vi "TempStrainRecord.vi"() -> ()   [LabVIEW 2024]
uses:
  <vilib>/Analysis/baseanly.llb/Mean (DBL).vi
  <vilib>/DAQmx/create/channels.llb/DAQmx Create Channel (AI-Temperature-Thermocouple).vi
  <vilib>/DAQmx/configure/trigger.llb/DAQmx Start Trigger (Digital Edge).vi
  <vilib>/Utility/TDMS File Viewer/NI_TDMS File Viewer.lvlib
  <vilib>/Analysis/NI_AALBase.lvlib
panel:
  in  "stop":bool
  out "status":bool
  out "DAQ error out":errorcluster caption="error out"
  out "Temp loop counter":i32
  out "mean 2":dbl format="%0.2f"
  out "mean 3":dbl format="%0.2f"
  out "mean 4":dbl format="%0.2f"
  out "mean 5":dbl format="%0.2f"
  out "data 5":dynamicdata(graph) caption="data"
  out "data 4":dynamicdata(graph) caption="data"
  out "mean 0":dbl format="%0.2f"
  out "data 3":dynamicdata(graph) caption="data"
  out "data 2":dynamicdata(graph) caption="data"
  out "data 1":dynamicdata(graph) caption="data"
  out "data 0":dynamicdata(graph) caption="data"
  out "mean 1":dbl format="%0.2f"
  out "Temperature TDMS error out":errorcluster
  out "TCP warning out":errorcluster
  out "TDMS Close error out":errorcluster
  out "TCP counter":i32
  out "Complete String after 'Bytes to read'":string
  out "Bytes to read (hex)":string
  out "Bytes to read (dec)":i32
  out "Qty of Optical Lines":string
  out "LineNumber":string
  out "Date":string
  out "OpticalLineNumber":string[](array[string])
  out "Qty of FBG's":string[](array[string])
  out "System Status":string[][](array[string])
  out "Peak Wavelengths":string[][](array[string])
  out "Peak Powers":string[][](array[string])
  out "Time":string
  in  "Address":string="127.0.0.1"
  in  "Port":u16=2055 min=1025 step=1
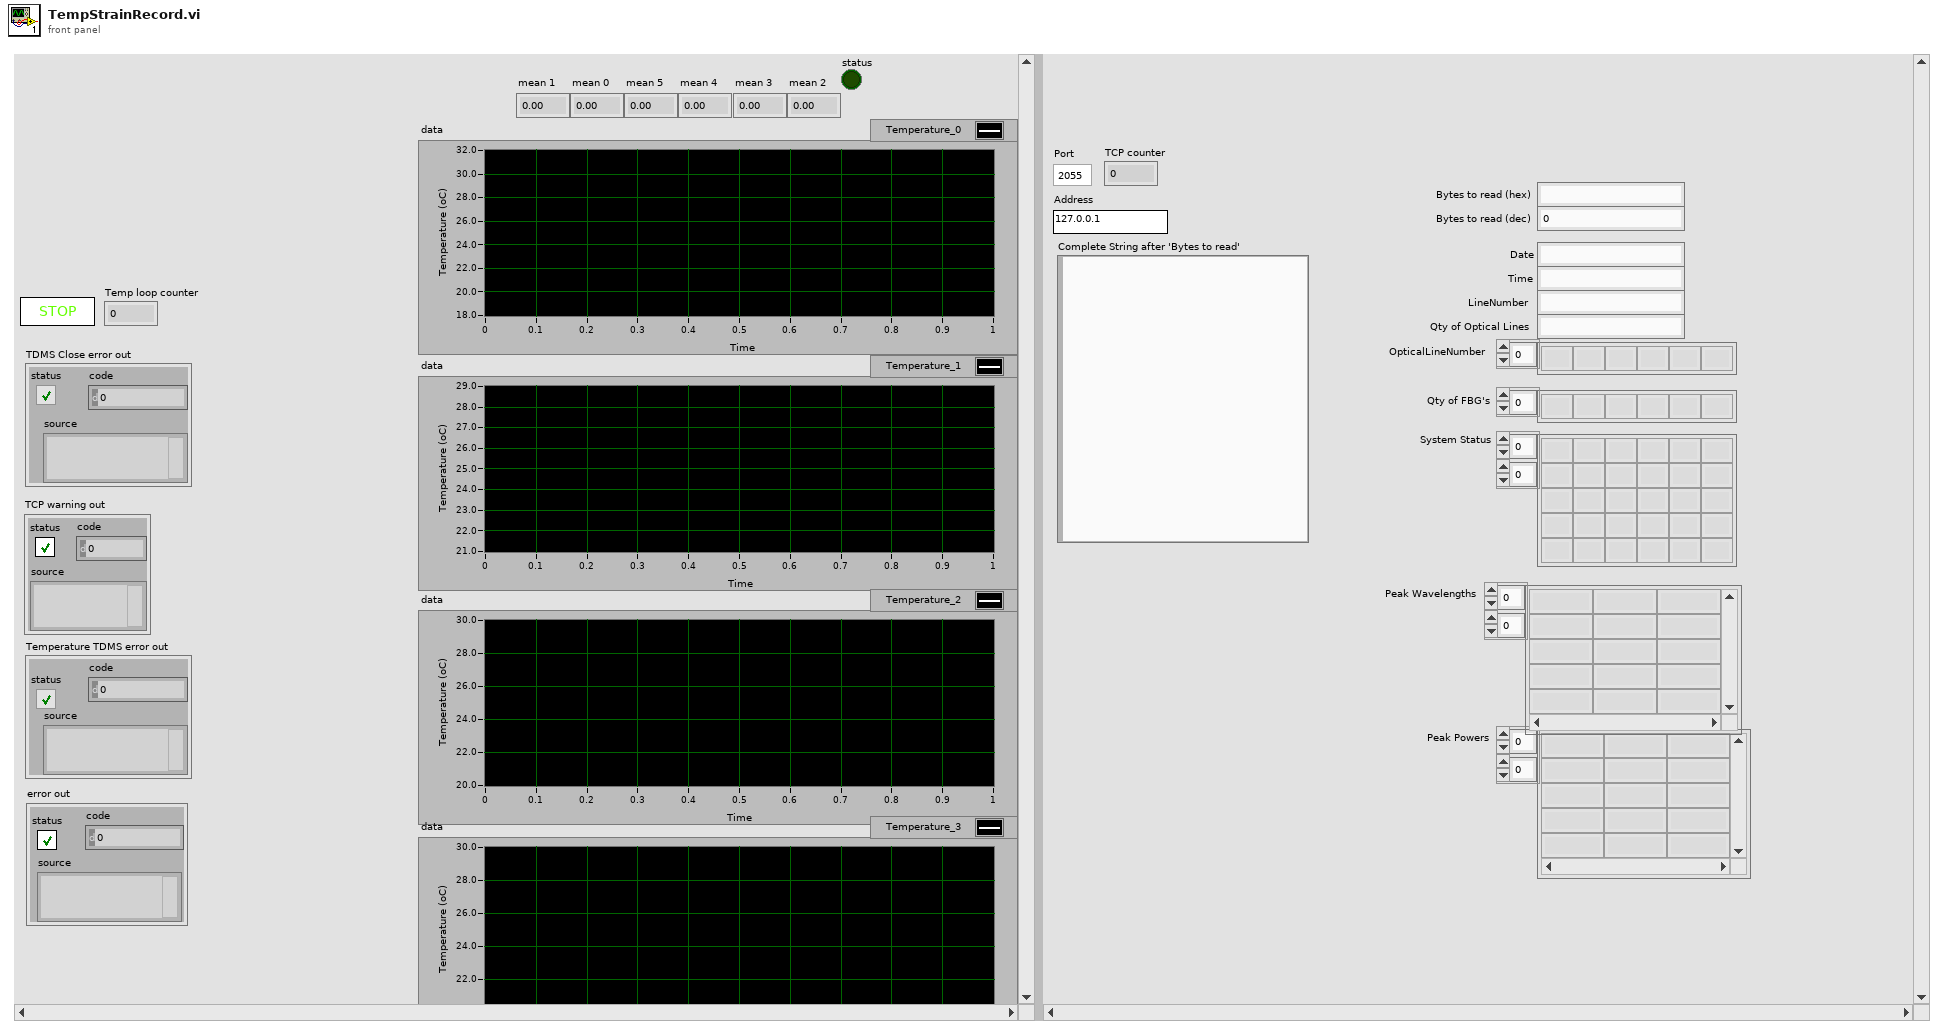
[diagram p1: front panel]
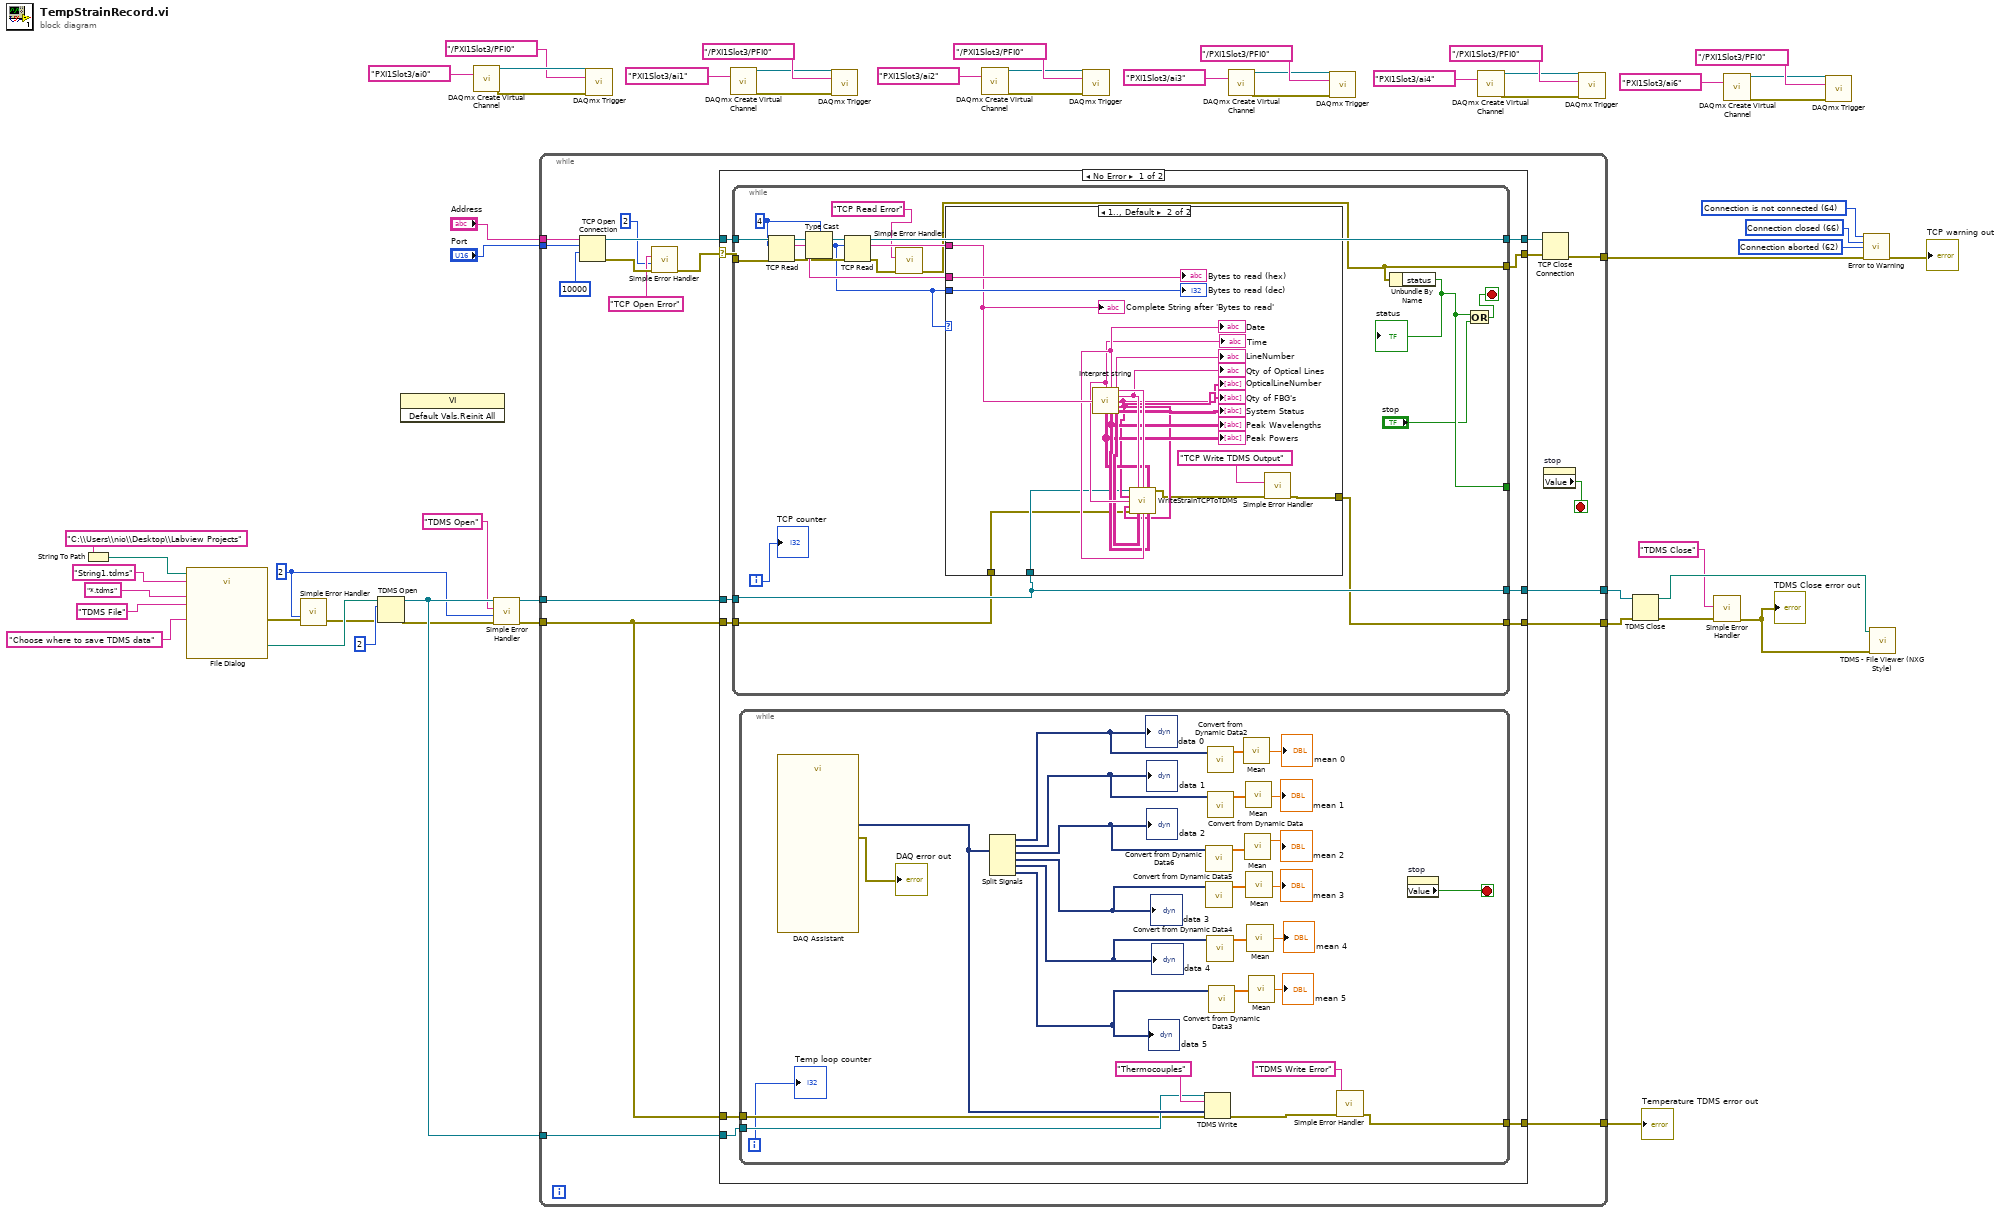
[diagram p0: block diagram]
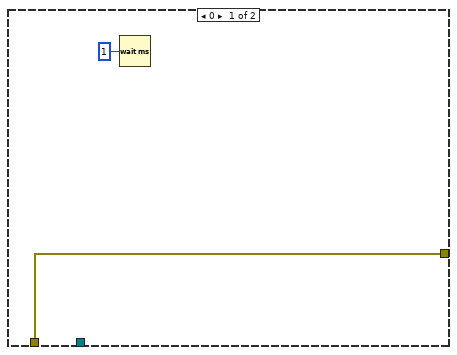
[diagram p2: hidden frame]
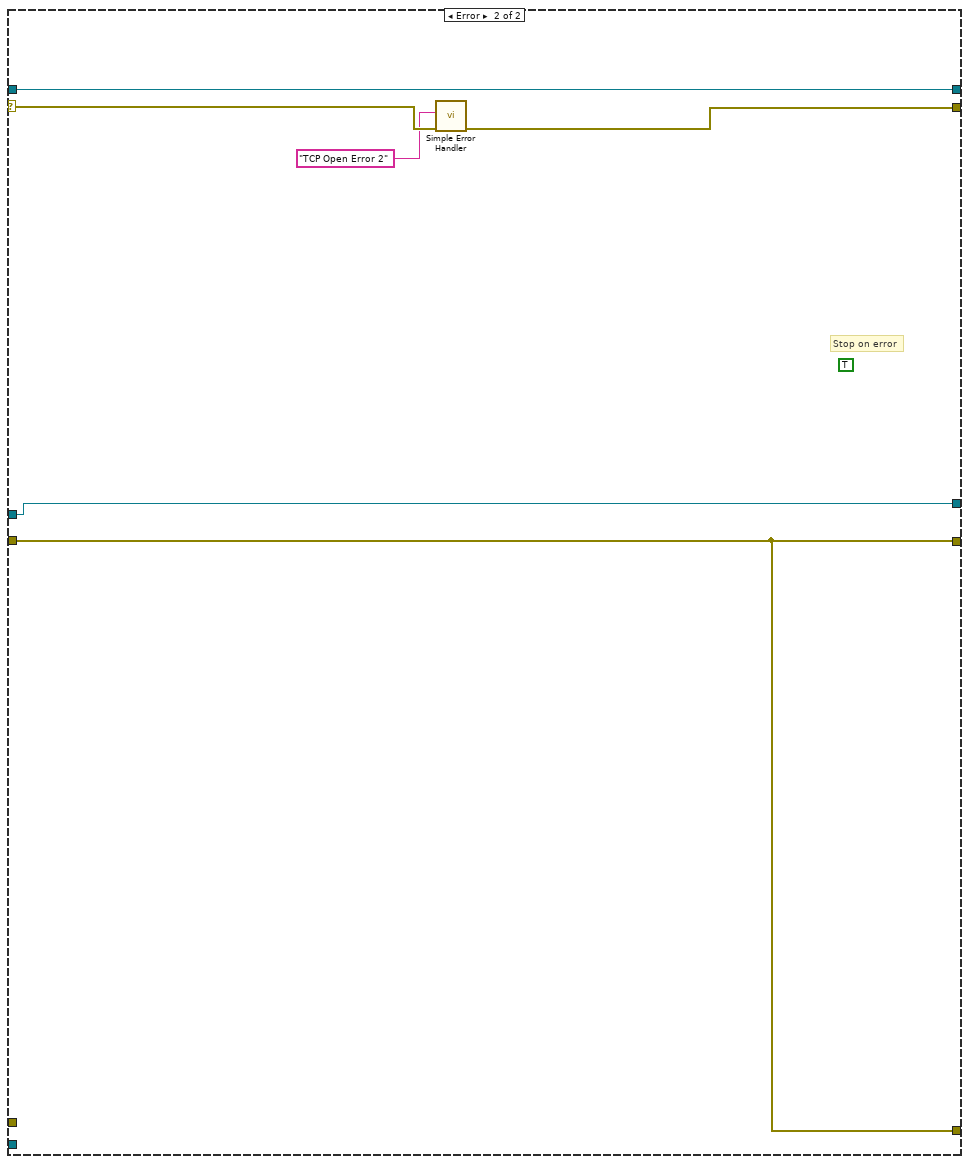
[diagram p3: hidden frame]
diagram:
  w1 = 2
  w23 = 62 items=["No Error", "Argument Error", "Memory Full", "Out of Zone", "End of File", "File Already Open", "Generic File IO Error", "File Not Found", "File Permission Error", "Disk Full", "Duplicate Path", "Too Many Files Open", "Not Enabled", "Resource File Not Found", "Cannot Add Resource", "Resource Not Found", "Image Not Found", "Image Memory Error", "Pen Does Not Exist", "Config Bad Type", "Config Token Not Found", "Config Parse Error", "Config Memory Error", "Bad External Code Format", "Bad External Code Offset", "External Code Not Present", "Null Window", "Destroy Window Mixup", "Null Menu", "Print Aborted", "Bad Print Record", "Print Driver Error", "Windows Error During Print", "Memory Error During Print", "Print Dialog Error", "Generic Print Error", "Invalid Device Refnum", "Device Not Found", "Device Parameter Error", "Device Unit Error", "Can't Open Device", "Device Call Aborted", "Generic Error", "Cancelled By User", "Object ID Too Low", "Object ID Too High", "Object Not In Heap", "Unknown Heap", "Bad DefProc ID", "DefProc Not In Table", "Message Out Of Range", "Null Method", "Unknown Message", "Manager Call Not Supported", "Bad address", "Connection In progress", "Connection timed out", "Connection is already in progress", "Network attribute not supported", "Network error", "Address in use", "System out of memory", "Connection aborted", "Connection refused", "Connection is not connected", "Connection is already connected", "Connection closed", "Initialize error (interapplication manager)", "Bad occurrence", "Wait on unbound occurrence handler", "Occurrence queue overflow", "Bad path", "Semaphore not signaled", "Unrecognized type (interapplication manager)"] ("1st Error to Convert")
  w24 = 66 items=["No Error", "Argument Error", "Memory Full", "Out of Zone", "End of File", "File Already Open", "Generic File IO Error", "File Not Found", "File Permission Error", "Disk Full", "Duplicate Path", "Too Many Files Open", "Not Enabled", "Resource File Not Found", "Cannot Add Resource", "Resource Not Found", "Image Not Found", "Image Memory Error", "Pen Does Not Exist", "Config Bad Type", "Config Token Not Found", "Config Parse Error", "Config Memory Error", "Bad External Code Format", "Bad External Code Offset", "External Code Not Present", "Null Window", "Destroy Window Mixup", "Null Menu", "Print Aborted", "Bad Print Record", "Print Driver Error", "Windows Error During Print", "Memory Error During Print", "Print Dialog Error", "Generic Print Error", "Invalid Device Refnum", "Device Not Found", "Device Parameter Error", "Device Unit Error", "Can't Open Device", "Device Call Aborted", "Generic Error", "Cancelled By User", "Object ID Too Low", "Object ID Too High", "Object Not In Heap", "Unknown Heap", "Bad DefProc ID", "DefProc Not In Table", "Message Out Of Range", "Null Method", "Unknown Message", "Manager Call Not Supported", "Bad address", "Connection In progress", "Connection timed out", "Connection is already in progress", "Network attribute not supported", "Network error", "Address in use", "System out of memory", "Connection aborted", "Connection refused", "Connection is not connected", "Connection is already connected", "Connection closed", "Initialize error (interapplication manager)", "Bad occurrence", "Wait on unbound occurrence handler", "Occurrence queue overflow", "Bad path", "Semaphore not signaled", "Unrecognized type (interapplication manager)"] ("1st Error to Convert")
  w25 = 64 items=["No Error", "Argument Error", "Memory Full", "Out of Zone", "End of File", "File Already Open", "Generic File IO Error", "File Not Found", "File Permission Error", "Disk Full", "Duplicate Path", "Too Many Files Open", "Not Enabled", "Resource File Not Found", "Cannot Add Resource", "Resource Not Found", "Image Not Found", "Image Memory Error", "Pen Does Not Exist", "Config Bad Type", "Config Token Not Found", "Config Parse Error", "Config Memory Error", "Bad External Code Format", "Bad External Code Offset", "External Code Not Present", "Null Window", "Destroy Window Mixup", "Null Menu", "Print Aborted", "Bad Print Record", "Print Driver Error", "Windows Error During Print", "Memory Error During Print", "Print Dialog Error", "Generic Print Error", "Invalid Device Refnum", "Device Not Found", "Device Parameter Error", "Device Unit Error", "Can't Open Device", "Device Call Aborted", "Generic Error", "Cancelled By User", "Object ID Too Low", "Object ID Too High", "Object Not In Heap", "Unknown Heap", "Bad DefProc ID", "DefProc Not In Table", "Message Out Of Range", "Null Method", "Unknown Message", "Manager Call Not Supported", "Bad address", "Connection In progress", "Connection timed out", "Connection is already in progress", "Network attribute not supported", "Network error", "Address in use", "System out of memory", "Connection aborted", "Connection refused", "Connection is not connected", "Connection is already connected", "Connection closed", "Initialize error (interapplication manager)", "Bad occurrence", "Wait on unbound occurrence handler", "Occurrence queue overflow", "Bad path", "Semaphore not signaled", "Unrecognized type (interapplication manager)"] ("1st Error to Convert")
  n1 = String To Path(string="C:\\Users\\nio\\Desktop\\Labview Projects") -> (path=w17:path)
  n2 = call "File Dialog"("start path"=w17, "prompt"="Choose where to save TDMS data", "default name"="String1.tdms", "pattern (all files)"="*.tdms", "pattern label"="TDMS File") -> ("selected path"=w51:path, "error out"=w15:errorcluster)  [unwired: 7 in, 2 out]
  n3 = call <vilib>:"Simple Error Handler.vi"("type of dialog (OK msg:1)"=w1, "error in (no error)"=w15) -> ("error out"=w14:errorcluster)  [unwired: 3 in, 4 out]
  n4 = TDMS Open(8:w14, 10:u32 2 ("milliseconds to wait"), 11:w51) -> (0:w10:errorcluster, 3:w20:refnum<k34>)  [unwired: 4 in]
  n5 = invoke class="VI" method="Default Vals.Reinit All"() -> ()  [unwired: 3 in, 3 out]
  n6 = call-poly <vilib>:"DAQmx Create Virtual Channel.vi"("physical channels"=tag "PXI1Slot3/ai0") -> ("task out"=w49:refnum<k21>, "error out"=w48:errorcluster)  [unwired: 13 in]
  n7 = call <vilib>:"Simple Error Handler.vi"("error source (\" \")"="TDMS Open", "type of dialog (OK msg:1)"=w1, "error in (no error)"=w10) -> ("error out"=w8:errorcluster)  [unwired: 2 in, 4 out]
  n8 = while {
    tunnel: [w68] -> w26
    tunnel: "Address" -> [w67]
    tunnel: "Port" -> [w66]
    tunnel: w20 -> [w64]
    tunnel: w20 -> [w63]
    tunnel: [w62] -> w19
    tunnel: [w61] -> w11
    tunnel: w8 -> [w55]
    tunnel: [w56] -> w4
    stop <- w54 stop-if-true
    n9 = TCP Open Connection(address=w67, remote port or service name=w66, timeout ms (60000)=10000) -> (connection ID=w69:refnum<k5>, error out=w60:errorcluster)  [unwired: 2 in]
    n10 = call <vilib>:"Simple Error Handler.vi"("error source (\" \")"="TCP Open Error", "type of dialog (OK msg:1)"=2, "error in (no error)"=w60) -> ("error out"=w59:errorcluster)  [unwired: 2 in, 4 out]
    n11 = case shown="No Error" w59 {
      selector: w59 -> [w79 w151]
      tunnel: [w82 w150] -> w71
      tunnel: [w81 w154] -> w70
      tunnel: w69 -> [w80 w154]
      tunnel: w64 -> [w74 _]
      tunnel: w63 -> [w78 w153]
      tunnel: [w77 w153] -> w62
      tunnel: [w76 w152] -> w61
      tunnel: w55 -> [w75 w152]
      tunnel: [w73 w152] -> w56
      tunnel: w55 -> [w72 _]
      frame No Error {
        n12 = while {
          tunnel: w79 -> [w126]
          tunnel: w80 -> [w127]
          tunnel: [w128] -> w81
          tunnel: [w114] -> w82
          tunnel: w78 -> [w120]
          tunnel: [w120] -> w77
          tunnel: [w119] -> w76
          tunnel: [w112] -> _
          tunnel: w75 -> [w118]
          i -> [w113]
          stop <- w115 stop-if-true
          w122 = 4
          n13 = TCP Read(connection ID=w127, bytes to read=w122, error in (no error)=w126) -> (connection ID out=w129:refnum<k5>, data out=w125:string, error out=w123:errorcluster)  [unwired: 2 in]
          n14 = Type Cast(type=w122, x=w125) -> (*(type *) &x=w121:i32)
          n15 = TCP Read(connection ID=w129, bytes to read=w121, error in (no error)=w123) -> (connection ID out=w128:refnum<k5>, data out=w124:string, error out=w117:errorcluster)  [unwired: 2 in]
          n16 = call <vilib>:"Simple Error Handler.vi"("error source (\" \")"="TCP Read Error", "error in (no error)"=w117) -> ("error out"=w114:errorcluster)  [unwired: 3 in, 4 out]
          n17 = case shown="1.., Default" w121 {
            tunnel: w125 -> [_ w148]
            tunnel: w124 -> [_ w146]
            tunnel: w121 -> [_ w147]
            tunnel: w120 -> [_ w136]
            tunnel: [w130 w134] -> w119
            tunnel: w118 -> [w130 w132]
            frame 0 {
              n18 = Wait (ms)(milliseconds to wait=u32 1) -> ()  [unwired: 1 out]
            }
            frame 1.., Default {
              n19 = call "Interpret string.vi"("Spreadsheet string"=w146) -> ("Time"=w144:string, "Date"=w145:string, "LineNumber"=w143:string, "Qty of Optical Lines"=w142:string, "OpticalLineNumber"=w137:string[], "Qty of FBG's"=w138:string[], "Peak Powers"=w139:string[][], "Peak Wavelengths"=w140:string[][], "System Status"=w141:string[][])  [unwired: 6 in]
              "Qty of Optical Lines" <- w142
              "LineNumber" <- w143
              "Date" <- w145
              "OpticalLineNumber" <- w137
              "Qty of FBG's" <- w138
              "System Status" <- w141
              "Peak Wavelengths" <- w140
              "Peak Powers" <- w139
              "Time" <- w144
              n20 = call "WriteStrainTCPToTDMS.vi"("TDMS In"=w136, "Qty of Optical Lines"=w142, "LineNumber"=w143, "Peak Powers"=w139, "OpticalLineNumber"=w137, "Time"=w144, "Qty of FBG's"=w138, "error in (no error)"=w132, "System Status"=w141, "Date"=w145, "Peak Wavelengths"=w140) -> ("tdms error out"=w135:errorcluster)  [unwired: 4 in]
              n21 = call <vilib>:"Simple Error Handler.vi"("error source (\" \")"="TCP Write TDMS Output", "error in (no error)"=w135) -> ("error out"=w134:errorcluster)  [unwired: 3 in, 4 out]
              "Complete String after 'Bytes to read'" <- w146
              "Bytes to read (hex)" <- w148
              "Bytes to read (dec)" <- w147
            }
          }
          n22 = Unbundle By Name(w114) -> ("status"=w112:bool)
          "status" <- w112
          n23 = Or(x=w112, y="stop") -> (x .or. y?=w115:bool)
          "TCP counter" <- w113
        }
        n24 = while {
          tunnel: w74 -> [w88]
          tunnel: [w87] -> w73
          tunnel: w72 -> [w86]
          i -> [w85]
          stop <- w83 stop-if-true
          n25 = call "DAQ Assistant"() -> ("data"=w108:dynamicdata, "error out"=→"DAQ error out":errorcluster)  [unwired: 17 in, 1 out]
          n26 = Split Signals(w108) -> (w96:dynamicdata, w93:dynamicdata, w105:dynamicdata, w106:dynamicdata, w107:dynamicdata, w109:dynamicdata)  [unwired: 6 in]
          "data 0" <- w96
          "data 1" <- w93
          "data 2" <- w105
          "data 3" <- w106
          "data 4" <- w107
          "data 5" <- w109
          n27 = TDMS Write(0:w88, 5:"Thermocouples" ("group name in (Untitled)"), 9:w108, 11:w86) -> (15:w110:errorcluster)  [unwired: 2 in, 3 out]
          n28 = call "Convert from Dynamic Data6"("Dynamic Data Type"=w105) -> ("Array"=w103:dbl[])  [unwired: 3 in]
          n29 = call "Convert from Dynamic Data5"("Dynamic Data Type"=w106) -> ("Array"=w101:dbl[])  [unwired: 3 in]
          n30 = call "Convert from Dynamic Data4"("Dynamic Data Type"=w107) -> ("Array"=w99:dbl[])  [unwired: 3 in]
          n31 = call "Convert from Dynamic Data2"("Dynamic Data Type"=w96) -> ("Array"=w94:dbl[])  [unwired: 3 in]
          n32 = call "Convert from Dynamic Data"("Dynamic Data Type"=w93) -> ("Array"=w91:dbl[])  [unwired: 3 in]
          n33 = call "Convert from Dynamic Data3"("Dynamic Data Type"=w109) -> ("Array"=w97:dbl[])  [unwired: 3 in]
          n34 = call-poly <vilib>:"Mean.vi"("X"=w94) -> ("mean"=→"mean 0":dbl)  [unwired: 1 out]
          n35 = call-poly <vilib>:"Mean.vi"("X"=w103) -> ("mean"=→"mean 2":dbl)  [unwired: 1 out]
          n36 = call-poly <vilib>:"Mean.vi"("X"=w91) -> ("mean"=→"mean 1":dbl)  [unwired: 1 out]
          n37 = call-poly <vilib>:"Mean.vi"("X"=w101) -> ("mean"=→"mean 3":dbl)  [unwired: 1 out]
          n38 = call-poly <vilib>:"Mean.vi"("X"=w99) -> ("mean"=→"mean 4":dbl)  [unwired: 1 out]
          n39 = call-poly <vilib>:"Mean.vi"("X"=w97) -> ("mean"=→"mean 5":dbl)  [unwired: 1 out]
          n40 = call <vilib>:"Simple Error Handler.vi"("error source (\" \")"="TDMS Write Error" ("group name in (Untitled)"), "error in (no error)"=w110) -> ("error out"=w87:errorcluster)  [unwired: 3 in, 4 out]
          n41 = property on="stop" class="Bool (strict)"() -> ("Value"=w83:bool)  [unwired: 2 in, 2 out]
          "Temp loop counter" <- w85
        }
      }
      frame Error {
        (unwired) TRUE
        # "Stop on error"
        n42 = call <vilib>:"Simple Error Handler.vi"("error source (\" \")"="TCP Open Error 2", "error in (no error)"=w151) -> ("error out"=w150:errorcluster)  [unwired: 3 in, 4 out]
      }
    }
    n43 = TCP Close Connection(connection ID=w70, error in (no error)=w71) -> (error out=w68:errorcluster)  [unwired: 1 in, 1 out]
    n44 = property on="stop" class="Bool (strict)"() -> ("Value"=w54:bool)  [unwired: 2 in, 2 out]
  }
  "Temperature TDMS error out" <- w4
  n45 = call-poly <vilib>:"DAQmx Trigger.vi"("task/channels in"=w49, "source"=tag "/PXI1Slot3/PFI0", "error in"=w48) -> ()  [unwired: 11 in, 2 out]
  n46 = call-poly <vilib>:"DAQmx Create Virtual Channel.vi"("physical channels"=tag "PXI1Slot3/ai1") -> ("task out"=w43:refnum<k21>, "error out"=w45:errorcluster)  [unwired: 13 in]
  n47 = call-poly <vilib>:"DAQmx Trigger.vi"("task/channels in"=w43, "source"=tag "/PXI1Slot3/PFI0", "error in"=w45) -> ()  [unwired: 11 in, 2 out]
  n48 = call-poly <vilib>:"DAQmx Create Virtual Channel.vi"("physical channels"=tag "PXI1Slot3/ai2") -> ("task out"=w39:refnum<k21>, "error out"=w41:errorcluster)  [unwired: 13 in]
  n49 = call-poly <vilib>:"DAQmx Trigger.vi"("task/channels in"=w39, "source"=tag "/PXI1Slot3/PFI0", "error in"=w41) -> ()  [unwired: 11 in, 2 out]
  n50 = call-poly <vilib>:"DAQmx Create Virtual Channel.vi"("physical channels"=tag "PXI1Slot3/ai3") -> ("task out"=w35:refnum<k21>, "error out"=w37:errorcluster)  [unwired: 13 in]
  n51 = call-poly <vilib>:"DAQmx Trigger.vi"("task/channels in"=w35, "source"=tag "/PXI1Slot3/PFI0", "error in"=w37) -> ()  [unwired: 11 in, 2 out]
  n52 = call-poly <vilib>:"DAQmx Create Virtual Channel.vi"("physical channels"=tag "PXI1Slot3/ai4") -> ("task out"=w31:refnum<k21>, "error out"=w33:errorcluster)  [unwired: 13 in]
  n53 = call-poly <vilib>:"DAQmx Trigger.vi"("task/channels in"=w31, "source"=tag "/PXI1Slot3/PFI0", "error in"=w33) -> ()  [unwired: 11 in, 2 out]
  n54 = TDMS Close(8:w11, 11:w19) -> (0:w7:errorcluster, 3:w21:path)
  n55 = call <vilib>:"Simple Error Handler.vi"("error source (\" \")"="TDMS Close", "error in (no error)"=w7) -> ("error out"=w6:errorcluster)  [unwired: 3 in, 4 out]
  "TDMS Close error out" <- w6
  n56 = call-poly <vilib>:"DAQmx Create Virtual Channel.vi"("physical channels"=tag "PXI1Slot3/ai6") -> ("task out"=w27:refnum<k21>, "error out"=w29:errorcluster)  [unwired: 13 in]
  n57 = call-poly <vilib>:"DAQmx Trigger.vi"("task/channels in"=w27, "source"=tag "/PXI1Slot3/PFI0", "error in"=w29) -> ()  [unwired: 11 in, 2 out]
  n58 = call <vilib>:"Error to Warning.vi"("1st Error to Convert"=w25, "2nd Error to Convert"=w24, "3rd Error to Convert"=w23, "error in"=w26) -> ("warning out"=→"TCP warning out":errorcluster)  [unwired: 11 in]
  n59 = call <vilib>:"TDMS - File Viewer (NXG Style).vi"("error in"=w6, "file in"=w21) -> ()  [unwired: 8 in, 2 out]
